vi "Set Multi.vi"(0 "Display State In":T1, 5 "Value":bool, 7 "First":bool, 9 "Container State":T2, 11 "error in (no error)":errorcluster) -> (4 "Display State Out":T1, 6 "mixed":bool, 15 "error out":errorcluster)   [LabVIEW 2015, in "KCheckbox.xctl"]
uses:
  KCheckbox.xctl
  <vilib>/_xctls/Container State.ctl
  State.ctl
  <vilib>/_xctls/XControlSupport.lvlib
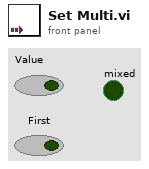
[diagram p1: front panel]
types:
  T1 = typedef "KCheckbox.xctl/State.ctl" = cluster{"mixed":bool, "Value":bool, "update":bool}
  T2 = typedef "XControlSupport.lvlib/Container State.ctl" = cluster{"Indicator?":bool, "Run Mode?":bool, " Refnum":refnum<vi>}
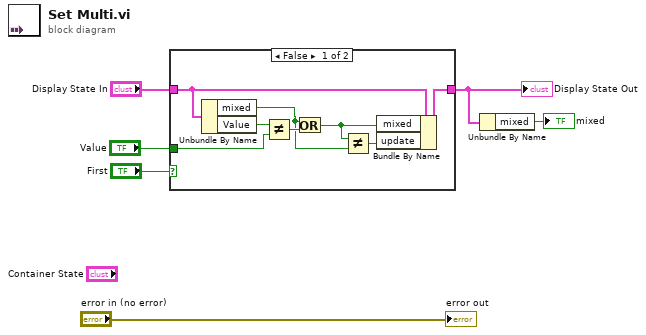
[diagram p0: block diagram]
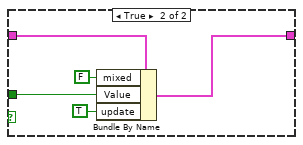
[diagram p2: hidden frame]
diagram:
  n1 = case shown="False" "First" {
    tunnel: "Display State In" -> [w14 w19]
    tunnel: [w10 w18] -> w2
    tunnel: "Value" -> [w12 w16]
    frame False {
      n2 = Unbundle By Name(w14) -> ("mixed"=w8:bool, "Value"=w13:bool)
      n3 = Not Equal?(x=w13, y=w12) -> (x != y?=w11:bool)
      n4 = Or(x=w8, y=w11) -> (x .or. y?=w7:bool)
      n5 = Not Equal?(x=w7, y=w8) -> (x != y?=w9:bool)
      n6 = Bundle By Name(cluster=w14, "mixed"=w7, "update"=w9) -> (w10:T1)
    }
    frame True {
      n7 = Bundle By Name(cluster=w19, "mixed"=FALSE, "Value"=w16, "update"=TRUE) -> (w18:T1)
    }
  }
  "Display State Out" <- w2
  n8 = Unbundle By Name(w2) -> ("mixed"=→"mixed":bool)
  "error out" <- "error in (no error)"
